vi "Normalize Identifier.vi"(10 "Identifier":string) -> (2 "Normalized Identifier":string)   [LabVIEW 2019, in "Instrument Manager.lvclass"]
uses:
  Instrument Manager.lvclass
  Instrument Manager.lvclass/Instrument Manager.ctl
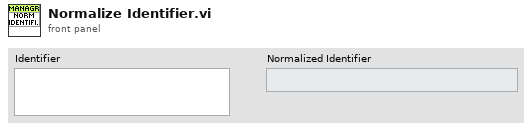
[diagram p1: front panel]
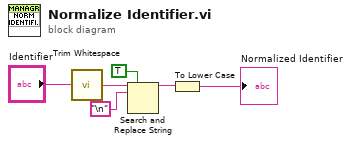
[diagram p0: block diagram]
diagram:
  n1 = call <vilib>:"Trim Whitespace.vi"("string"="Identifier") -> ("trimmed string"=w5:string)  [unwired: 1 in]
  n2 = Search and Replace String(replace all?=TRUE ("replace all? (F)"), input string=w5, search string="\n") -> (result string=w2:string)  [unwired: 5 in, 3 out]
  n3 = To Lower Case(string=w2) -> (all lower case string=→"Normalized Identifier":string)
